vi "Arm timer eating.vi"(8 "error in":errorcluster, 11 "Philosopher in":refnum<class "Philosopher.lvclass">) -> (0 "error out":errorcluster, 3 "Philosopher out":refnum<class "Philosopher.lvclass">)   [LabVIEW 2021, in "Philosopher.lvclass"]
uses:
  Philosopher.lvclass
  <vilib>/addons/_Workers/Library/Case Label.ctl
  <vilib>/addons/_Workers/Library/Workers.lvlib
  Timer/rqp_Start.ctl
  Timer/Timer.lvclass
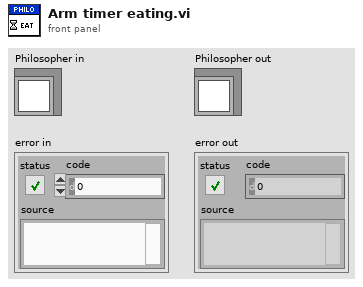
[diagram p1: front panel]
types:
  T1 = typedef "Timer.lvclass/rqp_Start.ctl" = cluster{"Timeout (ms)":i32, "# Copies":i32, "Response Case":T2}
  T2 = typedef "Workers.lvlib/Case Label.ctl" = string
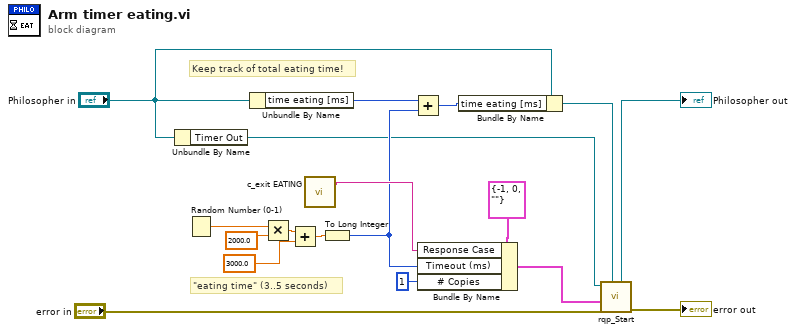
[diagram p0: block diagram]
diagram:
  # "Keep track of total eating time!"
  # "\"eating time\" (3..5 seconds)"
  n1 = Unbundle By Name("Philosopher in") -> ("Timer Out"=w1:refnum<class "Timer.lvclass">)
  n2 = Random Number (0-1)() -> (number: 0 to 1=w13:dbl)
  n3 = Unbundle By Name("Philosopher in") -> ("time eating [ms]"=w5:i32)
  n4 = Multiply(x=w13, y=2000.0) -> (x*y=w14:dbl)
  n5 = Add(x=w14, y=3000.0) -> (x+y=w12:dbl)
  n6 = call "c_exit EATING.vi"() -> ("Case Label"=w7:T2)  [unwired: 1 in]
  n7 = To Long Integer(number=w12) -> (32bit integer=w3:i32)
  n8 = Add(x=w5, y=w3) -> (x+y=w6:i32)
  n9 = Bundle By Name(cluster=T1 {"Timeout (ms)"=-1, "# Copies"=0, "Response Case"=""} ("Data in"), "Response Case"=w7, "Timeout (ms)"=w3, "# Copies"=1 ("# copies (0 = infinite repeat)")) -> (w15:T1)
  n10 = Bundle By Name(cluster="Philosopher in", "time eating [ms]"=w6) -> (w4:refnum<class "Philosopher.lvclass">)
  n11 = call "rqp_Start.vi"("Caller in"=w4, "error in"="error in", "Data in"=w15, "Timer In"=w1) -> ("error out"=→"error out":errorcluster, "dup Caller out"=→"Philosopher out":refnum<class "Philosopher.lvclass">)  [unwired: 5 in, 1 out]
